vi "Count Peaks (SubVI).vi"(7 "Done":bool, 8 "Increment":bool) -> (0 "Peak Count":u16)   [LabVIEW 2015]
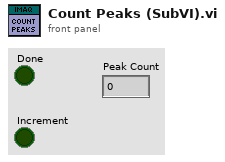
[diagram p1: front panel]
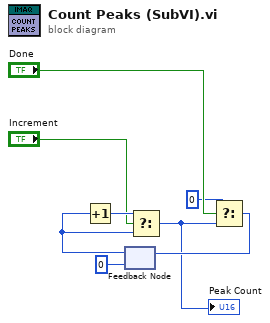
[diagram p0: block diagram]
diagram:
  n1 = feedback #1(u16 0 ("Count Out")) -> (w4:u16)
  n2 = Increment(x=w4) -> (x+1=w5:u16)
  n3 = Select(t=w5, s="Increment", f=w4) -> (s? t:f=w1:u16)
  "Peak Count" <- w1
  n4 = Select(t=u16 0, s="Done", f=w1) -> (s? t:f=w8:u16)
  n5 = feedback-in #1(w8) -> ()
